vi "Set Mode.vi"(8 "error in (no error)":errorcluster, 11 "TCS in":refnum<class "TCS.lvclass">) -> (0 "error out":errorcluster, 3 "TCS out":refnum<class "TCS.lvclass">)   [LabVIEW 2018, in "TCS.lvclass"]
uses:
  TCS.lvclass
  C:/Users/observer/Desktop/Sparc4GUI/SPARC4_GUI/Server/Server.lvclass
  Server/Server.lvclass/Server.ctl
  Server/Server.lvclass
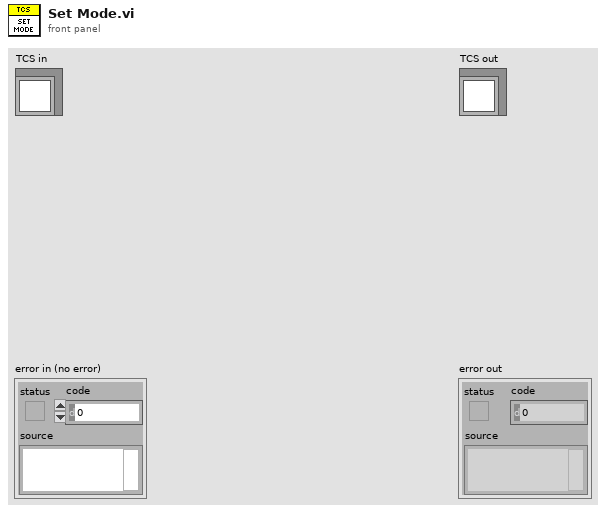
[diagram p1: front panel]
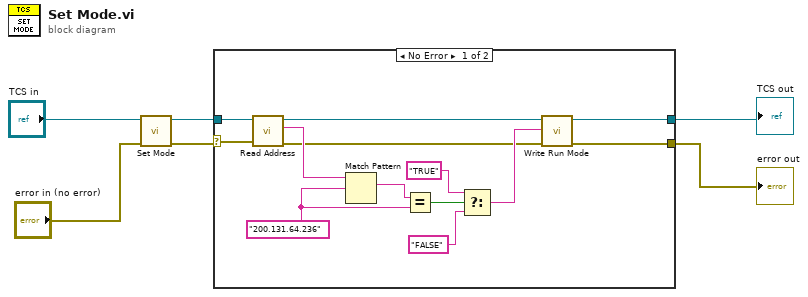
[diagram p0: block diagram]
diagram:
  n1 = call-parent "Set Mode.vi"("error in (no error)"="error in (no error)", "Server in"="TCS in") -> ("error out"=w4:errorcluster, "Server out"=w3:refnum<class "TCS.lvclass">)  [unwired: 8 in]
  n2 = case shown="No Error" w4 {
    selector: w4 -> [w18 w21]
    tunnel: w3 -> [w19 w20]
    tunnel: [w8 w21] -> w2
    tunnel: [w7 w20] -> w1
    frame No Error {
      w15 = "200.131.64.236" ("y")
      n3 = call "Read Address.vi"("error in (no error)"=w18, "Server in"=w19) -> ("error out"=w10:errorcluster, "Address"=w17:string, "Server out"=w9:refnum<class "TCS.lvclass">)  [unwired: 7 in]
      n4 = Match Pattern(string=w17, regular expression=w15) -> (match substring=w16:string)  [unwired: 1 in, 3 out]
      n5 = Equal?(x=w16, y=w15) -> (x = y?=w14:bool)
      n6 = Select(t="TRUE" ("y"), s=w14, f="FALSE" ("y")) -> (s? t:f=w11:string)
      n7 = call-dynamic "Write Run Mode.vi"("error in (no error)"=w10, "Run Mode"=w11, "Server in"=w9) -> ("error out"=w8:errorcluster, "Server out"=w7:refnum<class "TCS.lvclass">)  [unwired: 7 in]
    }
    frame Error {
    }
  }
  "error out" <- w2
  "TCS out" <- w1
